vi "Store Display State.vi"(6 "Data":T1={"t0"=timestamp(0 s since 1904-01-01), "dt"=0.0, "Y"=[]}, 7 "Operation In":T6, 8 "Error In (no Error) In":errorcluster, 9 "Container State In":T2 caption="Container State", 10 "Waveform State In":T3={"Show Axes"=FALSE, "Show Y=0"=FALSE, "Controls"={"Type"=enum."Sine", "Periods"=0.0, "Points"=0, "Offset"=0.0, "Amplitdue"=0.0, "Starting Phase"=0.0, "func"=""}, "Show Current Location"=FALSE, "Current Location"=0, "dt"=0.0, "t0"=timestamp(0 s since 1904-01-01)} caption="State", 11 "State In":T7 caption="State") -> (0 "Error Out":errorcluster, 2 "Waveform State Out":T3={"Show Axes"=FALSE, "Show Y=0"=FALSE, "Controls"={"Type"=enum."Sine", "Periods"=0.0, "Points"=0, "Offset"=0.0, "Amplitdue"=0.0, "Starting Phase"=0.0, "func"=""}, "Show Current Location"=FALSE, "Current Location"=0, "dt"=0.0, "t0"=timestamp(0 s since 1904-01-01)} caption="State", 3 "Display State Out":T7 caption="State", 4 "Data 2":T1 caption="Data")   [LabVIEW 2011, in "Waveform Control.xctl"]
uses:
  Waveform Control.xctl
  Function Types.ctl
  FP Controls.ctl
  Controls/State.ctl
  Controls/Waveform State.ctl
  <vilib>/_xctls/Container State.ctl
  <vilib>/_xctls/XControlSupport.lvlib
  Controls/Data.ctl
  Controls/Volatile State Ops.ctl
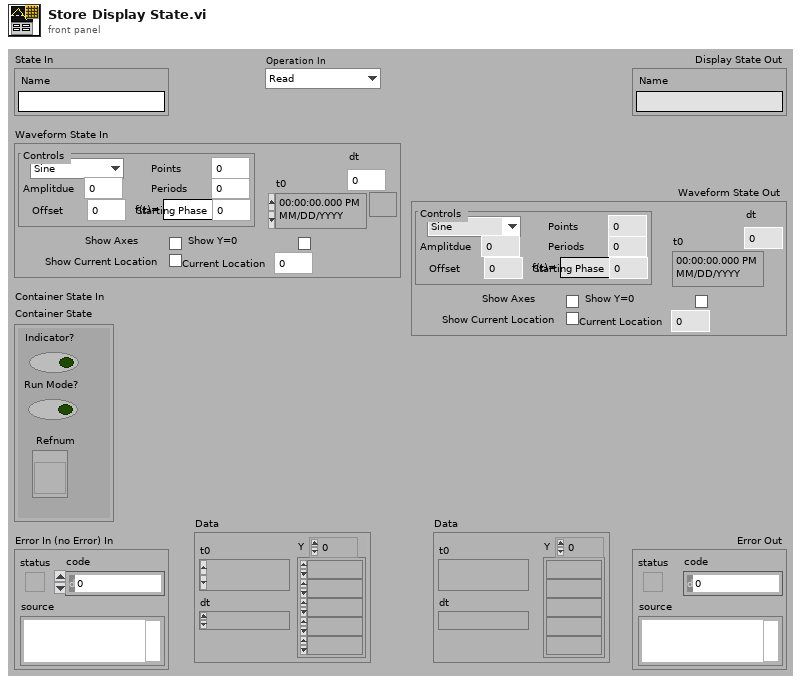
[diagram p1: front panel]
types:
  T1 = typedef "Waveform Control.xctl/Data.ctl" = waveform(dbl)
  T2 = typedef "XControlSupport.lvlib/Container State.ctl" = cluster{"Indicator?":bool, "Run Mode?":bool, " Refnum":refnum<vi>}
  T3 = typedef "Waveform Control.xctl/Waveform State.ctl" = cluster{"Show Axes":bool, "Show Y=0":bool, "Controls":T4, "Show Current Location":bool, "Current Location":i32, "dt":dbl, "t0":timestamp}
  T4 = typedef "Waveform Control.xctl/FP Controls.ctl" = cluster{"Type":T5, "Periods":dbl, "Points":i32, "Offset":dbl, "Amplitdue":dbl, "Starting Phase":dbl, "func":string}
  T5 = typedef "Waveform Control.xctl/Function Types.ctl" = enum16{"Level", "Sine", "Triangle", "Ramp", "Saw Tooth", "Square", "Function"}
  T6 = typedef "Waveform Control.xctl/Volatile State Ops.ctl" = enum16{"Read", "Write", "Update State from Data"}
  T7 = typedef "Waveform Control.xctl/State.ctl" = cluster{"Name":string}
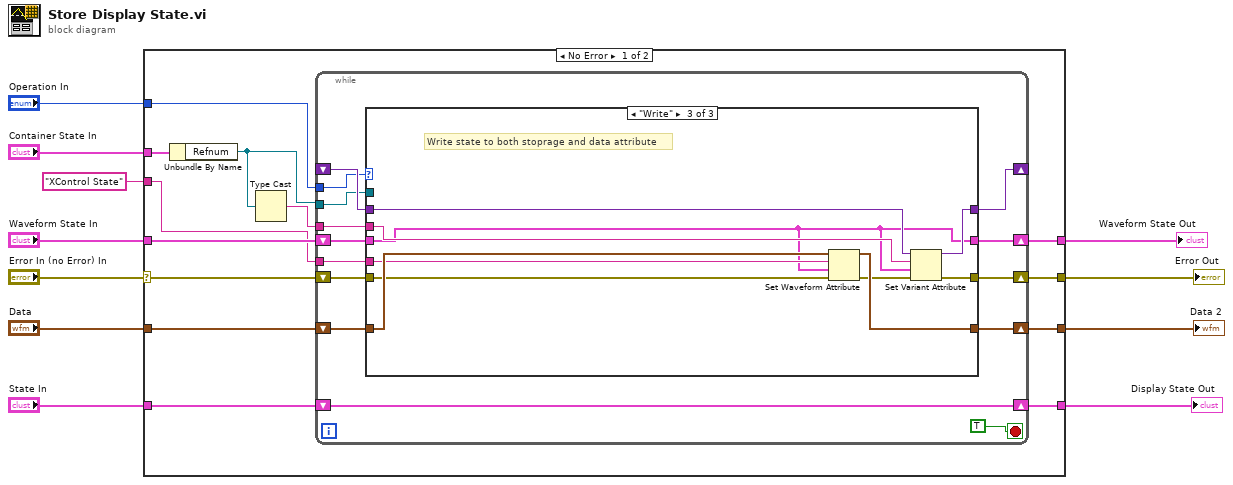
[diagram p0: block diagram]
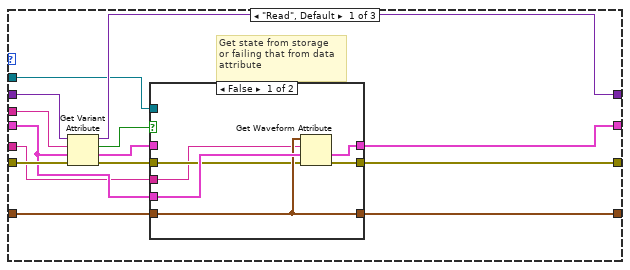
[diagram p2: hidden frame]
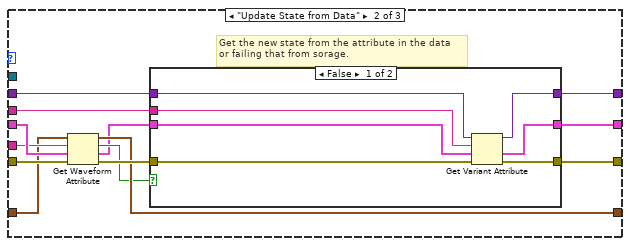
[diagram p4: hidden frame]
diagram:
  n1 = case shown="No Error" "Error In (no Error) In" {
    selector: "Error In (no Error) In" -> [w19 w98]
    tunnel: "Container State In" -> [w24 _]
    tunnel: "Operation In" -> [w22 _]
    tunnel: "Waveform State In" -> [w21 w97]
    tunnel: [w18 w98] -> w7
    tunnel: [w17 w97] -> w6
    tunnel: [w16 w96] -> w5
    tunnel: "State In" -> [w12 w96]
    tunnel: [w15 w95] -> w2
    tunnel: "Data" -> [w14 w95]
    tunnel: "XControl State" ("name") -> [w13 _]
    frame No Error {
      n2 = Unbundle By Name(w24) -> ("Refnum"=w20:refnum<vi>)
      n3 = Type Cast(x=w20) -> (*(type *) &x=w23:string)  [unwired: 1 out]
      n4 = while {
        shift-right: [w37] -> _
        shift-left: _ -> [w38]
        tunnel: w23 -> [w34]
        tunnel: w22 -> [w36]
        tunnel: w20 -> [w33]
        shift-right: [w25] -> w16
        shift-left: w12 -> [w25]
        shift-right: [w31] -> w18
        shift-left: w19 -> [w32]
        shift-right: [w30] -> w17
        shift-left: w21 -> [w35]
        shift-right: [w28] -> w15
        shift-left: w14 -> [w27]
        tunnel: w13 -> [w26]
        stop <- TRUE stop-if-true
        n5 = case shown="\"Write\"" w36 {
          tunnel: w38 -> [w52 w74 w94]
          tunnel: [w51 w73 w93] -> w37
          tunnel: w35 -> [w45 w71 w87]
          tunnel: w34 -> [w50 w72 w92]
          tunnel: w33 -> [w48 _ _]
          tunnel: w32 -> [w47 w69 w86]
          tunnel: [w44 w67 w91] -> w31
          tunnel: [w43 w62 w87] -> w30
          tunnel: [w41 w65 w89] -> w28
          tunnel: w27 -> [w40 w66 w90]
          tunnel: w26 -> [w39 w70 w88]
          frame "Read", Default {
            # "Get state from storage\nor failing that from data\nattribute"
            n6 = Get Variant Attribute(Variant=w52, name=w50, default value (empty Variant)=w45, error in=w47) -> (duplicate Variant=w51:variant, found=w49:bool, value=w42:T3, error out=w46:errorcluster)
            n7 = case shown="False" w49 {
              tunnel: w48 -> [_ _]
              tunnel: w46 -> [w54 w61]
              tunnel: w45 -> [w58 _]
              tunnel: [w57 w60] -> w43
              tunnel: [w56 w61] -> w44
              tunnel: w42 -> [_ w60]
              tunnel: [w55 w59] -> w41
              tunnel: w40 -> [w55 w59]
              tunnel: w39 -> [w53 _]
              frame False {
                n8 = Get Waveform Attribute(4:w54, 5:w58, 6:w53, 7:w55) -> (0:w56:errorcluster, 1:w57:T3)  [unwired: 2 out]
              }
              frame True {
              }
            }
          }
          frame "Update State from Data" {
            # "Get the new state from the attribute in the data\nor failing that from sorage."
            n9 = Get Waveform Attribute(4:w69, 5:w71, 6:w70, 7:w66) -> (0:w68:errorcluster, 1:w63:T3, 2:w64:bool, 3:w65:T1)
            n10 = case shown="False" w64 {
              tunnel: w74 -> [w81 w82]
              tunnel: [w80 w82] -> w73
              tunnel: w72 -> [w79 _]
              tunnel: w63 -> [w78 w83]
              tunnel: w68 -> [w77 w84]
              tunnel: [w76 w84] -> w67
              tunnel: [w75 w83] -> w62
              frame False {
                n11 = Get Variant Attribute(Variant=w81, name=w79, default value (empty Variant)=w78, error in=w77) -> (duplicate Variant=w80:variant, value=w75:T3, error out=w76:errorcluster)  [unwired: 1 out]
              }
              frame True {
              }
            }
          }
          frame "Write" {
            # "Write state to both stoprage and data attribute"
            n12 = Set Waveform Attribute(4:w86, 5:w87, 6:w88, 7:w90) -> (0:w85:errorcluster, 3:w89:T1)  [unwired: 1 out]
            n13 = Set Variant Attribute(Variant=w94, name=w92, value=w87, error in=w85) -> (Variant out=w93:variant, error out=w91:errorcluster)  [unwired: 1 out]
          }
        }
      }
    }
    frame Error {
    }
  }
  "Error Out" <- w7
  "Display State Out" <- w5
  "Waveform State Out" <- w6
  "Data 2" <- w2
